vi "KH TURCK ETHERNETIP RFID Global.vi"() -> ()   [LabVIEW 2017]
uses:
  KH TURCK ETHERNETIP TDef Enum RFID User Command.ctl
  KH TURCK ETHERNETIP TDefCluster TURCK RFID.ctl
  KH TURCK ETHERNETIP TDef Enum RFID Act Command.ctl
panel:
  in  "Tab Control 2":enum32{"RFID0", "RFID1", "Allgemein"}(tab)
  out "ErrorWriting0":bool[](array[boolean])
  out "WritingSuccessfull0":bool[](array[boolean])
  in  "RFID 0 LS Array":T1[](array[typedef])
  out "Error 0Array":bool[](array[boolean])
  out "BusyFinished 0Array":bool[](array[boolean])
  in  "UserCommand0Array":T3[](array[typedef])
  out "ErrorWriting1":bool[](array[boolean])
  out "WritingSuccessfull1":bool[](array[boolean])
  in  "RFID 1 LS Array":T1[](array[typedef])
  out "Error 1Array":bool[](array[boolean])
  out "BusyFinished 1Array":bool[](array[boolean])
  in  "UserCommand1Array":T3[](array[typedef])
  in  "Timeout":dbl=5.0
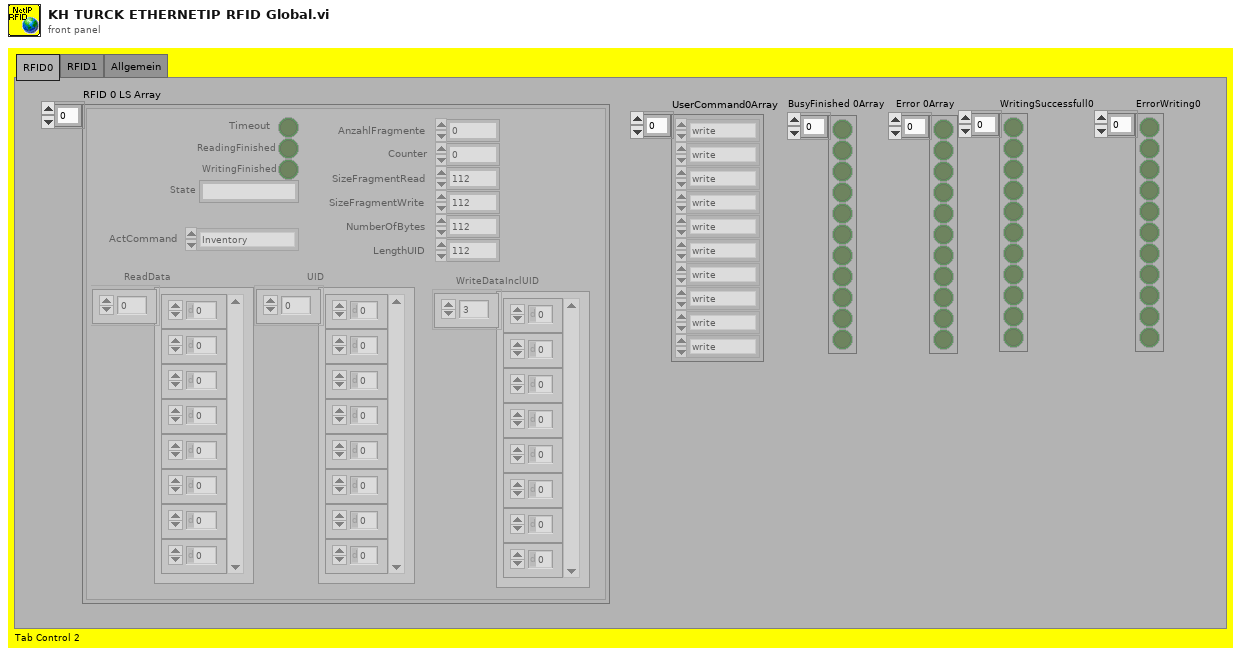
[diagram p1: front panel]
types:
  T1 = typedef "KH TURCK ETHERNETIP TDefCluster TURCK RFID.ctl" = cluster{"NumberOfBytes":i32, "State":string, "Counter":i32, "ReadData":u8[], "AnzahlFragmente":i32, "WritingFinished":bool, "ReadingFinished":bool, "UID":u8[], "ActCommand":T2, "SizeFragmentRead":i32, "LengthUID":u16, "WriteDataInclUID":u8[], "Timeout":bool, "SizeFragmentWrite":i32}
  T2 = typedef "KH TURCK ETHERNETIP TDef Enum RFID Act Command.ctl" = enum16{"read", "write", "idle", "Inventory", ""}
  T3 = typedef "KH TURCK ETHERNETIP TDef Enum RFID User Command.ctl" = enum16{"read", "write", "idle", "inventory"}
diagram:
